vi "navX Example v2.vi"() -> ()   [LabVIEW 2014]
uses:
  <vilib>/Rock Robotics/SystemInterfaces/i2clib/i2c_bus.ctl
  navX Library v2/IO/Open/navX Open I2C.vi
  navX Library v2/navX Library v2.lvlib
panel:
  in  "stop":bool
  out "Local Registry":u8[](array[numeric])
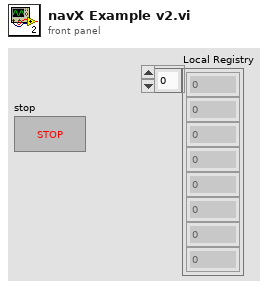
[diagram p1: front panel]
types:
  T1 = typedef "i2c_bus.ctl" = enum16{"I2C On-Board", "I2C MXP", "Invalid"}
  T2 = typedef "navX Library v2.lvlib/navX Device TypeDef.ctl" = cluster{"Interface":cluster{"Protocol":T3, "Update Rate (4Hz-60Hz)":u8, "navX Open TypeDef":variant}, "Notify Packet":refnum<notifier>, "Loop VI Refnum":refnum<vi>}
  T3 = typedef "navX Library v2.lvlib/navX Protocol TypeDef.ctl" = enum16{"SERIAL", "I2C", "SPI"}
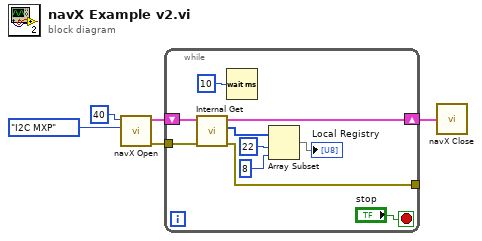
[diagram p0: block diagram]
diagram:
  n1 = call-poly "navX Open.vi"("I2C Bus"=i2c_bus."I2C MXP", "Update Rate (4Hz-60Hz)"=u8 40) -> ("error out"=w4:errorcluster, "navX Device"=w5:T2)  [unwired: 8 in]
  n2 = while {
    shift-right: [w13] -> w3
    shift-left: w5 -> [w15]
    tunnel: w4 -> [w14]
    tunnel: [w12] -> _
    stop <- "stop" stop-if-true
    n3 = call "Internal Get.vi"("error in (no error)"=w14, "navX Device"=w15) -> ("error out"=w12:errorcluster, "Local Registry"=w9:u8[], "navX Device"=w13:T2)  [unwired: 7 in]
    n4 = Wait (ms)(milliseconds to wait=u32 10) -> ()  [unwired: 1 out]
    n5 = Array Subset(array=w9, index=22, length=8 ("index")) -> (→"Local Registry":u8[])
  }
  n6 = call "navX Close.vi"("navX Device"=w3) -> ()
